vi "getSiteName.vi"(10 "Array":bool[](array[boolean])) -> (2 "String":string)   [LabVIEW 2012]
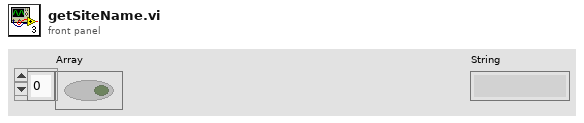
[diagram p1: front panel]
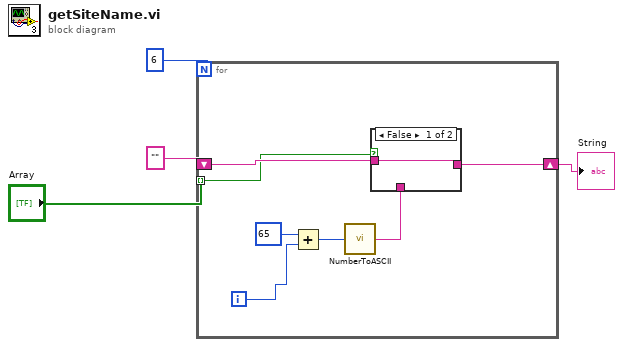
[diagram p0: block diagram]
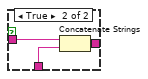
[diagram p2: hidden frame]
diagram:
  n1 = for {
    N: 6 -> [_]
    tunnel: "Array" -> [w5] mode=indexing
    shift-right: [w9] -> w2
    shift-left: "" -> [w10]
    i -> [w11]
    n2 = Add(x=65, y=w11) -> (x+y=w7:i32)
    n3 = call "NumberToASCII.vi"("number"=w7) -> ("ASCII"=w6:string)
    n4 = case shown="False" w5 {
      tunnel: w10 -> [w12 w15]
      tunnel: [w12 w14] -> w9
      tunnel: w6 -> [_ w13]
      frame False {
      }
      frame True {
        n5 = Concatenate Strings(w15, w13) -> (w14:string)
      }
    }
  }
  "String" <- w2
